vi "TC110.vi"(7 "Function":T3=enum."Read command", 8 "Error in":errorcluster, 10 "Settings in":T2) -> (0 "Error out":errorcluster, 1 "Status_string":string, 2 "Settings out":T2, 3 "output cluster":T1)   [LabVIEW 2018]
uses:
  clt/_ctl_PC_function_TC110.ctl
  clt/_ctl_PC_TurboSettings.ctl
  Public/Turbopumps/PV Operating adjustment - Cluster.ctl
  Pfeiffer Vacuum.lvlib
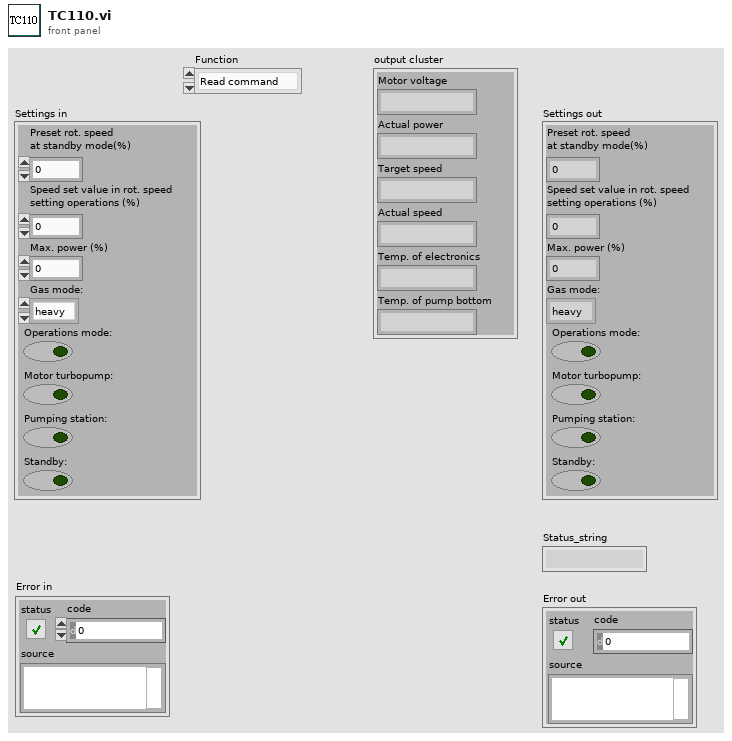
[diagram p1: front panel]
types:
  T1 = cluster{"Motor voltage":string, "Actual power":string, "Target speed":string, "Actual speed":string, "Temp. of electronics":string, "Temp. of pump bottom":string}
  T2 = typedef "_ctl_PC_TurboSettings.ctl" = cluster{"Preset rot. speed \nat standby mode(%)":dbl, "Speed set value in rot. speed \nsetting operations (%)":dbl, "Max. power (%)":dbl, "Gas mode: ":enum16{"heavy", "light", "helium"}, "Operations mode: ":bool, "Motor turbopump: ":bool, "Pumping station: ":bool, "Standby: ":bool}
  T3 = typedef "_ctl_PC_function_TC110.ctl" = enum16{"Initialisation", "Read status", "Write command", "Read command", "Close"}
  T4 = typedef "Pfeiffer Vacuum.lvlib/PV Operating adjustment - Cluster.ctl" = cluster{"Parameter":u16, "Parameter\nread only<->describe":bool, "off<->on":bool, "Rotation speed set value\nin rot. speed setting\noperations [%]":dbl, "Preset rotation Speed\nat Standby mode (%)":dbl, "maximum power\nsetpoint [%]":i32, "Gas mode":u16}
  T5 = enum16{"temperature inverter [°C] (324)", "temperature electronic [°C] (326)", "temperature pump bottom [°C] (330)", "temperature bearing [°C] (342)", "temperature motor [°C] (346)", "temperature rotor [°C] (384)"}
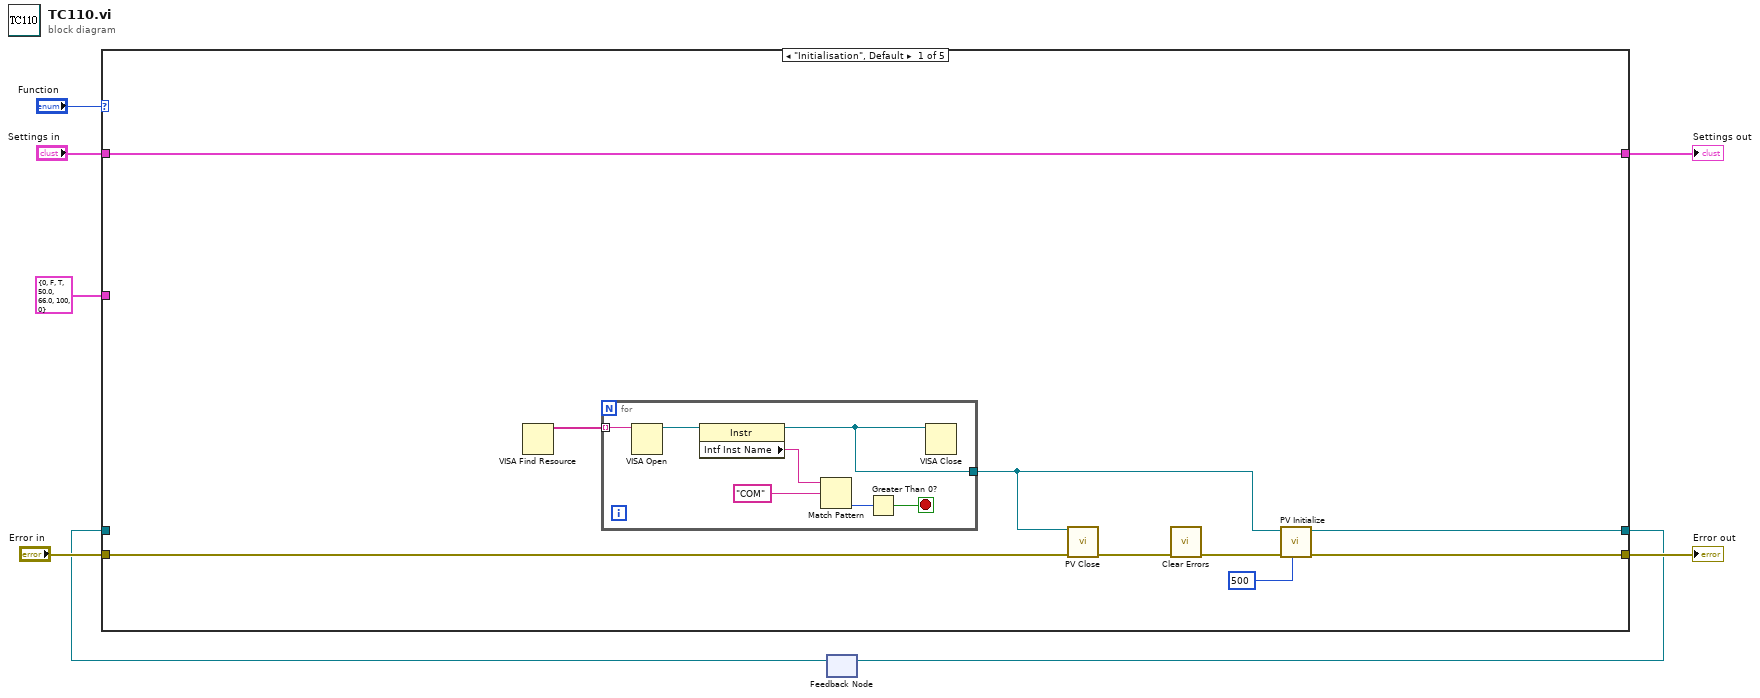
[diagram p0: block diagram]
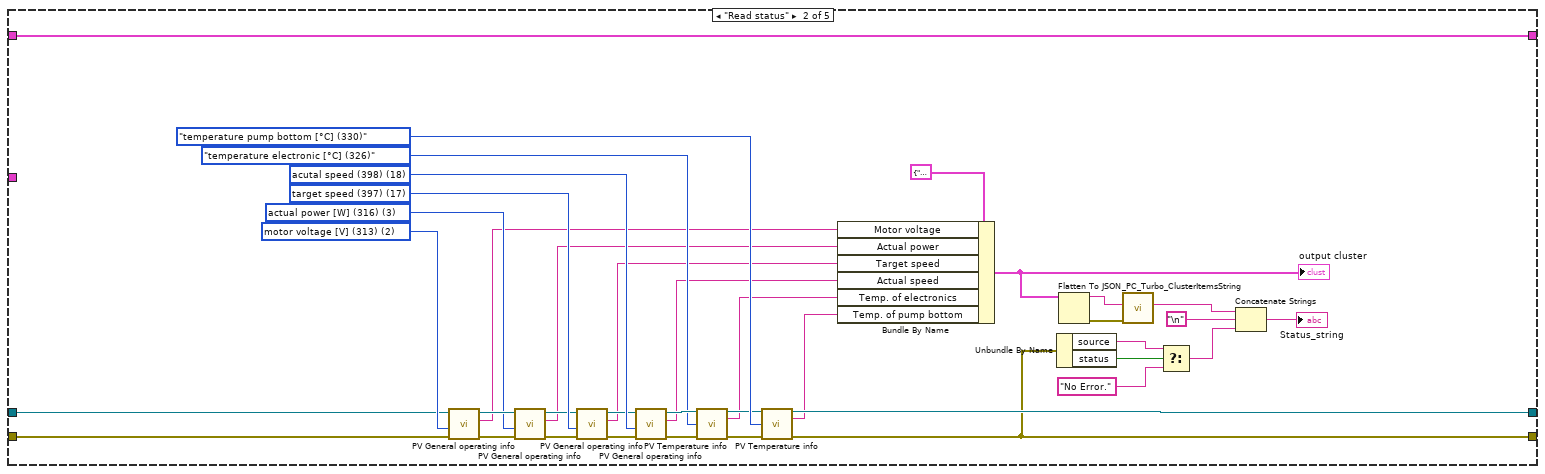
[diagram p2: hidden frame]
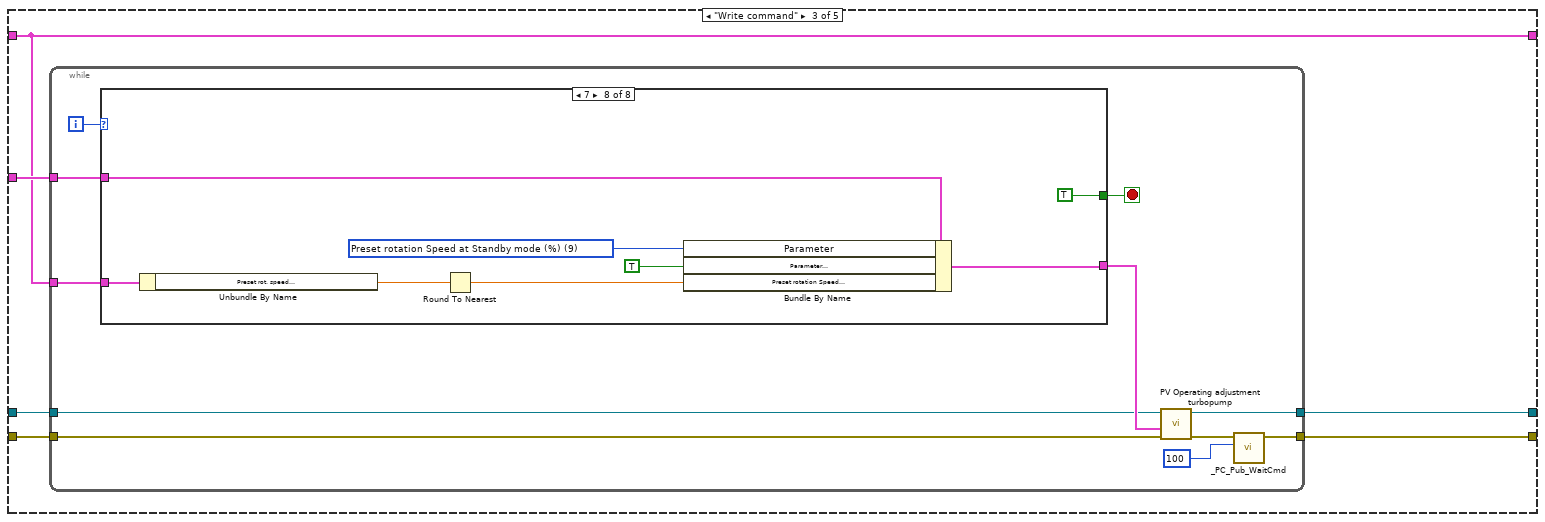
[diagram p3: hidden frame]
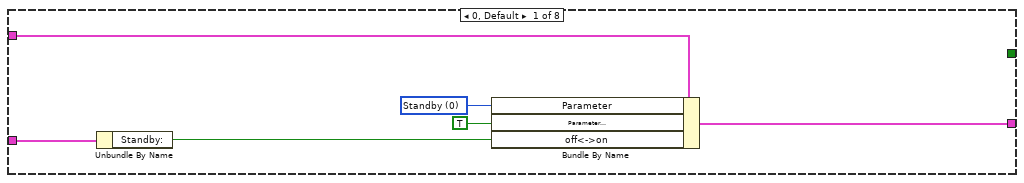
[diagram p4: hidden frame]
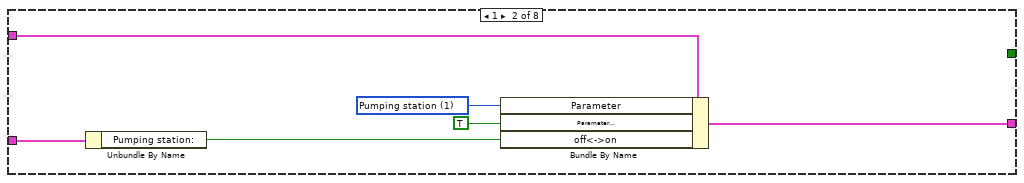
[diagram p5: hidden frame]
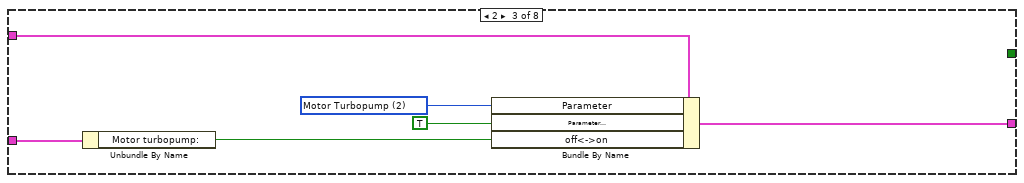
[diagram p6: hidden frame]
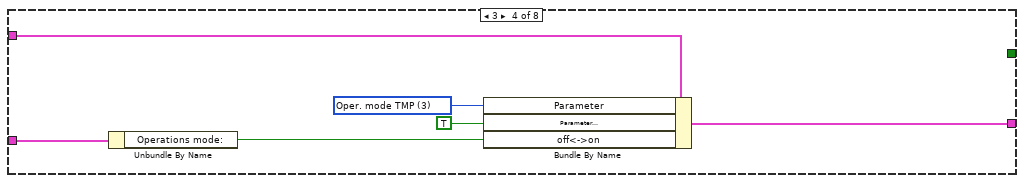
[diagram p7: hidden frame]
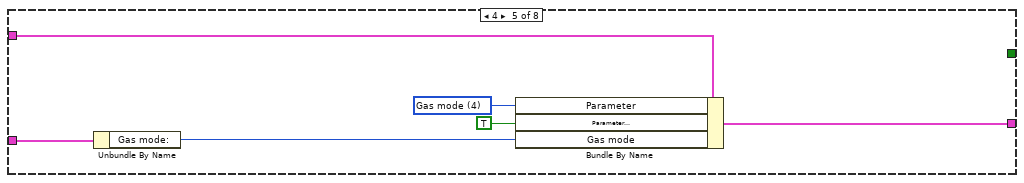
[diagram p8: hidden frame]
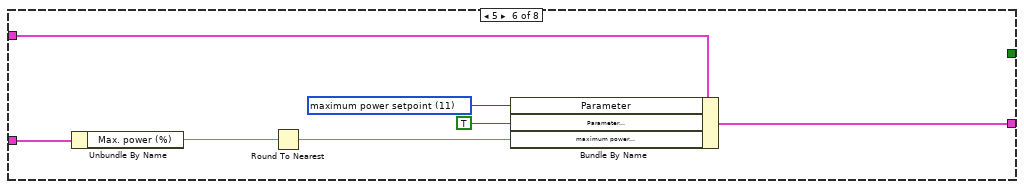
[diagram p9: hidden frame]
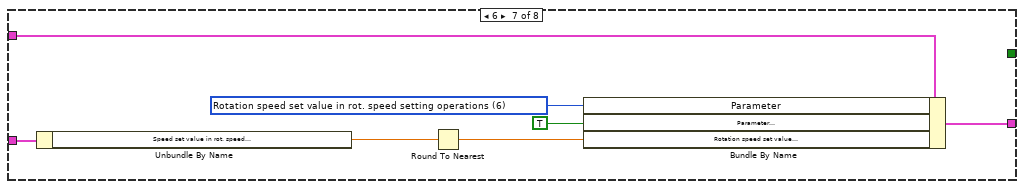
[diagram p10: hidden frame]
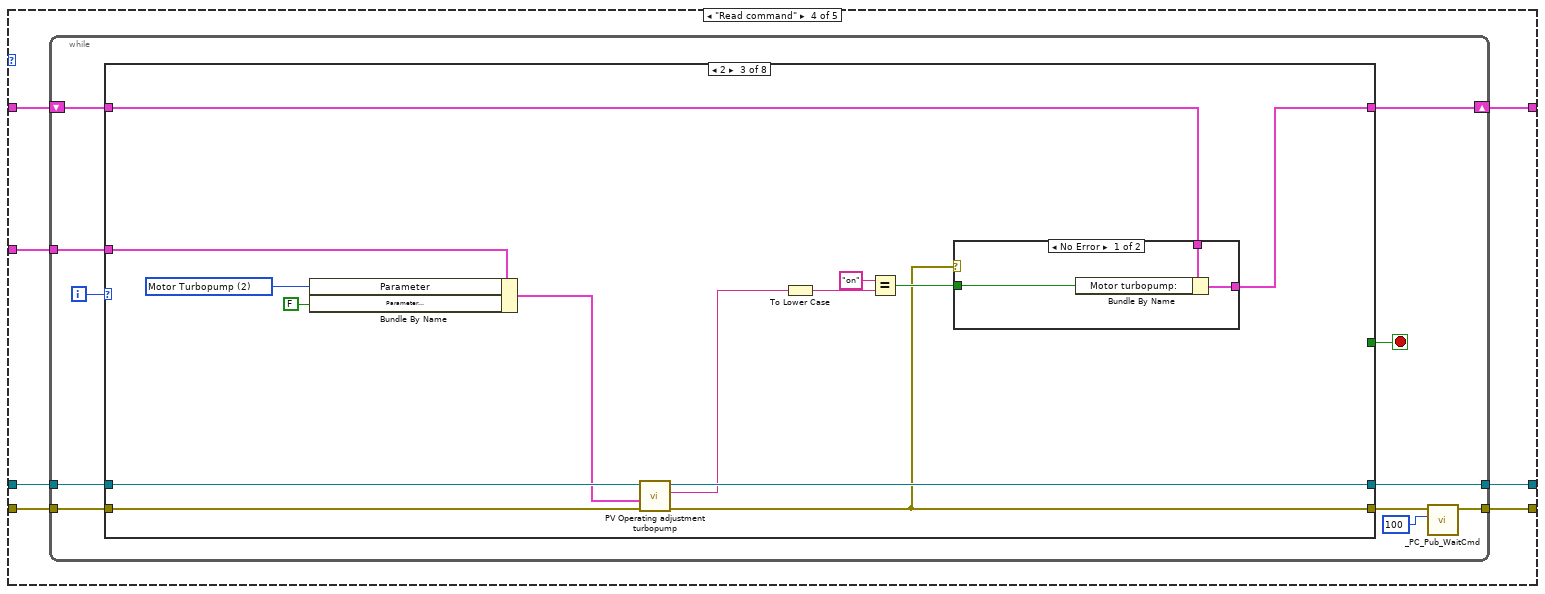
[diagram p11: hidden frame]
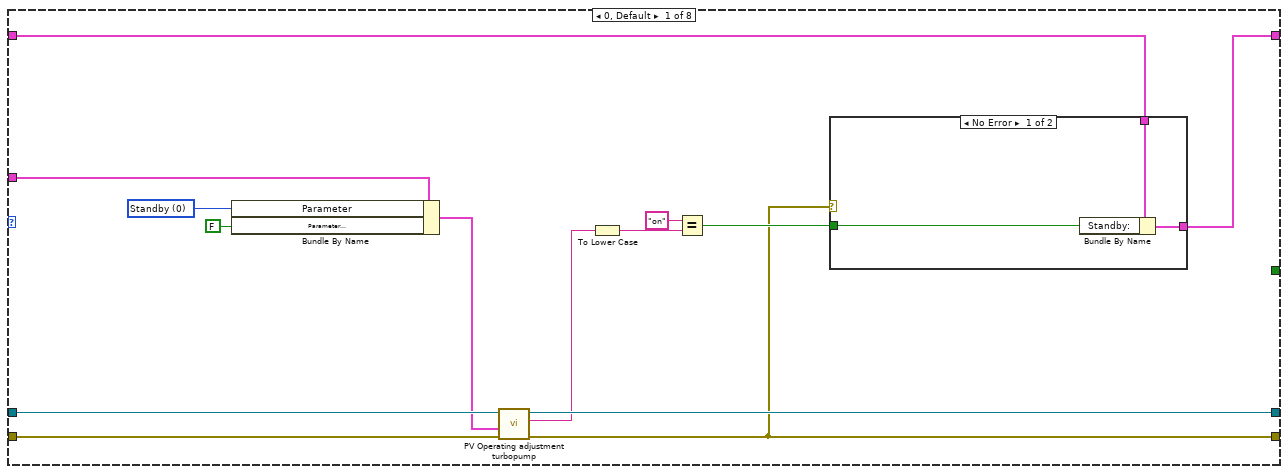
[diagram p12: hidden frame]
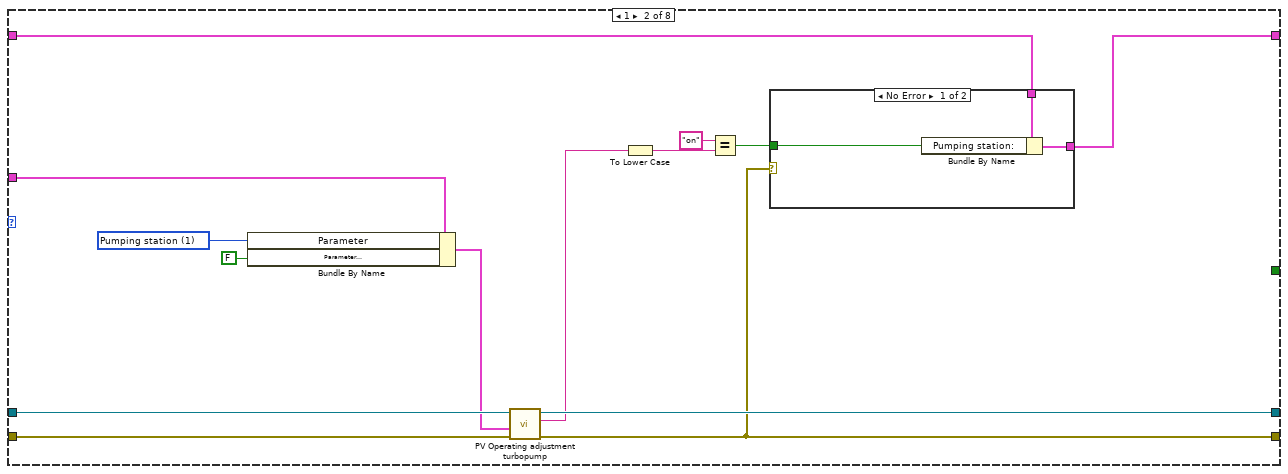
[diagram p14: hidden frame]
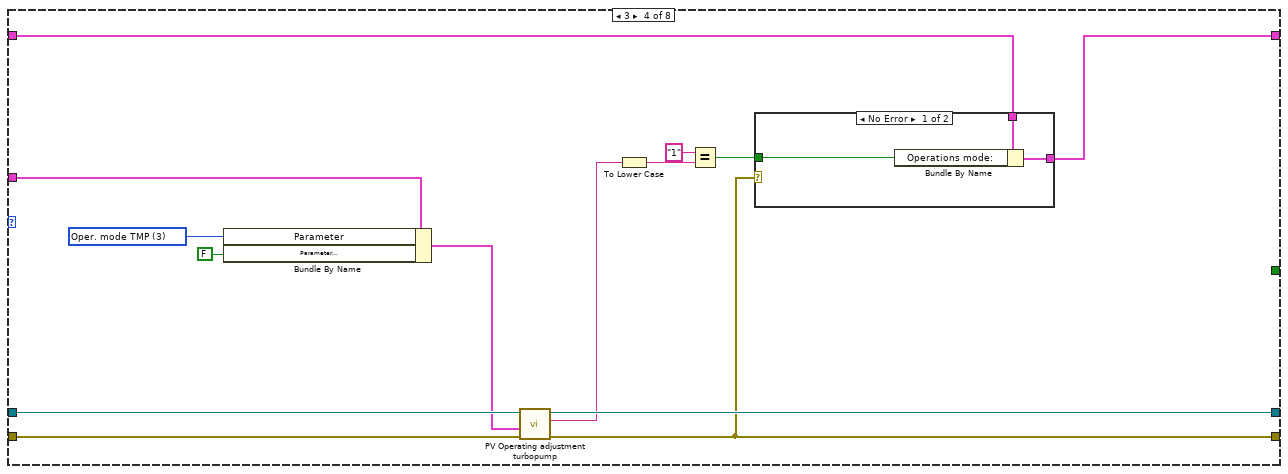
[diagram p17: hidden frame]
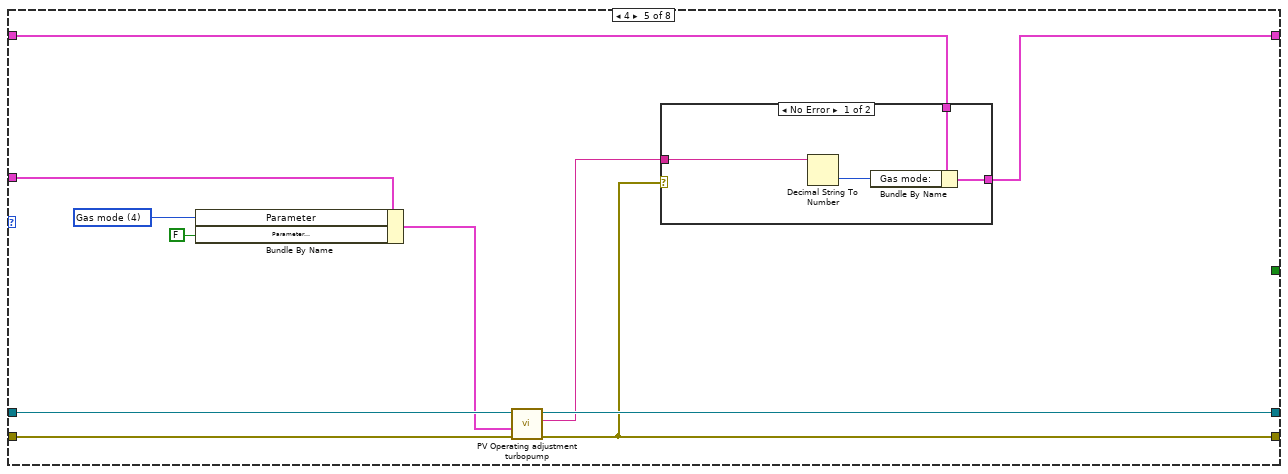
[diagram p19: hidden frame]
diagram:
  n1 = feedback #1() -> (w6:refnum<visa-resource-name>)  [unwired: 1 in]
  n2 = case shown="\"Initialisation\", Default" "Function" {
    tunnel: "Error in" -> [w13 w26 w66 w136 w291]
    tunnel: [w17 w42 w64 w133 _] -> w1
    tunnel: w6 -> [_ w27 w67 w137 w292]
    tunnel: [w16 w35 w65 w134 w290] -> w5
    tunnel: "Settings in" -> [w14 w25 w63 w135 w289]
    tunnel: T4 {"Parameter"=0, "Parameter\nread only<->describe"=FALSE, "off<->on"=TRUE, "Rotation speed set value\nin rot. speed setting\noperations [%]"=50.0, "Preset rotation Speed\nat Standby mode (%)"=66.0, "maximum power\nsetpoint [%]"=100, "Gas mode"=0} ("Operating adjustment - Cluster") -> [_ _ w68 w138 _]
    tunnel: [w14 w25 w63 w132 w289] -> w2
    frame "Initialisation", Default {
      n3 = VISA Find Resource() -> (3:w10:string[])  [unwired: 3 in, 2 out]
      n4 = for {
        tunnel: w10 -> [w24] mode=indexing
        tunnel: [w18] -> w9
        stop <- w20 stop-if-true
        n5 = VISA Open(VISA resource name=w24) -> (VISA resource name=w23:refnum<visa-resource-name>)  [unwired: 4 in, 1 out]
        n6 = property class="Instr"(reference=w23) -> (reference out=w18:refnum<visa-resource-name>, "Intf Inst Name"=w22:string)  [unwired: 1 in, 1 out]
        n7 = Match Pattern(string=w22, regular expression="COM") -> (offset past match=w19:i32)  [unwired: 1 in, 3 out]
        n8 = Greater Than 0?(x=w19) -> (x > 0?=w20:bool)
        n9 = VISA Close(VISA resource name=w18) -> ()  [unwired: 1 in, 1 out]
      }
      n10 = call "PV Close.vi"("VISA session"=w9, "error in (no error)"=w13) -> ("error out"=w12:errorcluster)  [unwired: 13 in]
      n11 = call <vilib>:"Clear Errors.vi"("error in (no error)"=w12) -> ("error out"=w11:errorcluster)  [unwired: 5 in, 1 out]
      n12 = call "PV Initialize.vi"("Timeout Value"=u32 500, "error in (no error)"=w11, "VISA session in"=w9) -> ("error out"=w16:errorcluster, "VISA session out"=w17:refnum<visa-resource-name>)  [unwired: 7 in]
    }
    frame "Read status" {
      w58 = u16 18 items=["nominal speed [Hz] (default) (315)", "intermediate circut current [A] (310)", "motor voltage [V] (313)", "actual power [W] (316)", "operating hours pump [h] (311)", "operating hours drive [h] (314)", "pump cycles (read only) (319)", "status oil sensor (read only) (301)", "speed switchpoint attained (read only) (302)", "overtemperature drive (read only) (304)", "overtemperature pump (read only) (305)", "target speed attained (read only) (306)", "pump accelerates (read only) (307) ", "controlled by remote (300)", "motor phase current [A] (317)", "acceleration / deceleration [rm/s] (336)", "hardware version controller (354)", "target speed (397)", "acutal speed (398)", "nominal speed (399)", "software version control unit (read only) (352)"] ("Parameter")
      w59 = u16 17 items=["nominal speed [Hz] (default) (315)", "intermediate circut current [A] (310)", "motor voltage [V] (313)", "actual power [W] (316)", "operating hours pump [h] (311)", "operating hours drive [h] (314)", "pump cycles (read only) (319)", "status oil sensor (read only) (301)", "speed switchpoint attained (read only) (302)", "overtemperature drive (read only) (304)", "overtemperature pump (read only) (305)", "target speed attained (read only) (306)", "pump accelerates (read only) (307) ", "controlled by remote (300)", "motor phase current [A] (317)", "acceleration / deceleration [rm/s] (336)", "hardware version controller (354)", "target speed (397)", "acutal speed (398)", "nominal speed (399)", "software version control unit (read only) (352)"] ("Parameter")
      w60 = u16 3 items=["nominal speed [Hz] (default) (315)", "intermediate circut current [A] (310)", "motor voltage [V] (313)", "actual power [W] (316)", "operating hours pump [h] (311)", "operating hours drive [h] (314)", "pump cycles (read only) (319)", "status oil sensor (read only) (301)", "speed switchpoint attained (read only) (302)", "overtemperature drive (read only) (304)", "overtemperature pump (read only) (305)", "target speed attained (read only) (306)", "pump accelerates (read only) (307) ", "controlled by remote (300)", "motor phase current [A] (317)", "acceleration / deceleration [rm/s] (336)", "hardware version controller (354)", "target speed (397)", "acutal speed (398)", "nominal speed (399)", "software version control unit (read only) (352)"] ("Parameter")
      w62 = u16 2 items=["nominal speed [Hz] (default) (315)", "intermediate circut current [A] (310)", "motor voltage [V] (313)", "actual power [W] (316)", "operating hours pump [h] (311)", "operating hours drive [h] (314)", "pump cycles (read only) (319)", "status oil sensor (read only) (301)", "speed switchpoint attained (read only) (302)", "overtemperature drive (read only) (304)", "overtemperature pump (read only) (305)", "target speed attained (read only) (306)", "pump accelerates (read only) (307) ", "controlled by remote (300)", "motor phase current [A] (317)", "acceleration / deceleration [rm/s] (336)", "hardware version controller (354)", "target speed (397)", "acutal speed (398)", "nominal speed (399)", "software version control unit (read only) (352)"] ("Parameter")
      n13 = call "PV General operating info.vi"("error in (no error)"=w26, "Parameter"=w62, "VISA session"=w27) -> ("error out"=w55:errorcluster, "response (data)"=w45:string, "dup VISA session"=w61:refnum<visa-resource-name>)  [unwired: 6 in]
      n14 = call "PV General operating info.vi"("error in (no error)"=w55, "Parameter"=w60, "VISA session"=w61) -> ("error out"=w54:errorcluster, "response (data)"=w39:string, "dup VISA session"=w57:refnum<visa-resource-name>)  [unwired: 6 in]
      n15 = call "PV General operating info.vi"("error in (no error)"=w54, "Parameter"=w59, "VISA session"=w57) -> ("error out"=w53:errorcluster, "response (data)"=w40:string, "dup VISA session"=w56:refnum<visa-resource-name>)  [unwired: 6 in]
      n16 = call "PV General operating info.vi"("error in (no error)"=w53, "Parameter"=w58, "VISA session"=w56) -> ("error out"=w49:errorcluster, "response (data)"=w44:string, "dup VISA session"=w52:refnum<visa-resource-name>)  [unwired: 6 in]
      n17 = call "PV Temperature info.vi"("VISA session"=w52, "Parameter"=T5."temperature electronic [°C] (326)", "error in (no error)"=w49) -> ("dup VISA session"=w48:refnum<visa-resource-name>, "response (data)"=w43:string, "error out"=w47:errorcluster)  [unwired: 10 in]
      n18 = call "PV Temperature info.vi"("VISA session"=w48, "Parameter"=T5."temperature pump bottom [°C] (330)", "error in (no error)"=w47) -> ("dup VISA session"=w42:refnum<visa-resource-name>, "response (data)"=w41:string, "error out"=w35:errorcluster)  [unwired: 10 in]
      n19 = Bundle By Name(cluster=T1 {"Motor voltage"="", "Actual power"="", "Target speed"="", "Actual speed"="", "Temp. of electronics"="", "Temp. of pump bottom"=""}, "Motor voltage"=w45, "Actual power"=w39, "Target speed"=w40, "Actual speed"=w44, "Temp. of electronics"=w43, "Temp. of pump bottom"=w41) -> (w38:T1)
      "output cluster" <- w38
      n20 = Unbundle By Name(w35) -> ("source"=w33:string, "status"=w34:bool)
      n21 = Flatten To JSON(anything=w38) -> (JSON string=w37:string, 11:w36:errorcluster)  [unwired: 2 in]
      n22 = call "_PC_Turbo_ClusterItemsString.vi"("error in (no error)"=w36, "JSON string"=w37) -> ("result string"=w31:string)  [unwired: 8 in, 1 out]
      n23 = Select(t=w33, s=w34, f="No Error.") -> (s? t:f=w29:string)
      n24 = Concatenate Strings(w31, "\n" ("string"), w29) -> (→"Status_string":string)
    }
    frame "Write command" {
      n25 = while {
        tunnel: w63 -> [w79]
        tunnel: w67 -> [w74]
        tunnel: w66 -> [w73]
        tunnel: [w70] -> w65
        tunnel: w68 -> [w78]
        tunnel: [w72] -> w64
        i -> [w77]
        stop <- w76 stop-if-true
        n26 = case shown="7" w77 {
          tunnel: w79 -> [w83 w89 w95 w101 w107 w114 w121 w129]
          tunnel: w78 -> [w85 w91 w97 w103 w109 w116 w123 w131]
          tunnel: [_ _ _ _ _ _ _ TRUE] -> w76
          tunnel: [w80 w86 w92 w98 w104 w110 w117 w124] -> w75
          frame 0, Default {
            w81 = u16 0 items=[" Standby", " Pumping station", " Motor Turbopump", " Oper. mode TMP", " Gas mode", " Operating mode drive unit", " Rotation speed set value in rot. speed setting operations", " Set rotation speed TMP [Hz] (read only)", " Actual rotation speed TMP [Hz] (read only)", " Preset rotation Speed at Standby mode (%)", " Max. rotations speed ", " maximum power setpoint"] ("Parameter")
            n27 = Unbundle By Name(w83) -> ("Standby:"=w82:bool)
            n28 = Bundle By Name(cluster=w85, "Parameter"=w81, "Parameter\nread only<->describe"=TRUE ("Parameter\nread only<->describe"), "off<->on"=w82) -> (w80:T4)
          }
          frame 1 {
            w87 = u16 1 items=[" Standby", " Pumping station", " Motor Turbopump", " Oper. mode TMP", " Gas mode", " Operating mode drive unit", " Rotation speed set value in rot. speed setting operations", " Set rotation speed TMP [Hz] (read only)", " Actual rotation speed TMP [Hz] (read only)", " Preset rotation Speed at Standby mode (%)", " Max. rotations speed ", " maximum power setpoint"] ("Parameter")
            n29 = Unbundle By Name(w89) -> ("Pumping station:"=w88:bool)
            n30 = Bundle By Name(cluster=w91, "Parameter"=w87, "Parameter\nread only<->describe"=TRUE ("Parameter\nread only<->describe"), "off<->on"=w88) -> (w86:T4)
          }
          frame 2 {
            w93 = u16 2 items=[" Standby", " Pumping station", " Motor Turbopump", " Oper. mode TMP", " Gas mode", " Operating mode drive unit", " Rotation speed set value in rot. speed setting operations", " Set rotation speed TMP [Hz] (read only)", " Actual rotation speed TMP [Hz] (read only)", " Preset rotation Speed at Standby mode (%)", " Max. rotations speed ", " maximum power setpoint"] ("Parameter")
            n31 = Unbundle By Name(w95) -> ("Motor turbopump:"=w94:bool)
            n32 = Bundle By Name(cluster=w97, "Parameter"=w93, "Parameter\nread only<->describe"=TRUE ("Parameter\nread only<->describe"), "off<->on"=w94) -> (w92:T4)
          }
          frame 3 {
            w99 = u16 3 items=[" Standby", " Pumping station", " Motor Turbopump", " Oper. mode TMP", " Gas mode", " Operating mode drive unit", " Rotation speed set value in rot. speed setting operations", " Set rotation speed TMP [Hz] (read only)", " Actual rotation speed TMP [Hz] (read only)", " Preset rotation Speed at Standby mode (%)", " Max. rotations speed ", " maximum power setpoint"] ("Parameter")
            n33 = Unbundle By Name(w101) -> ("Operations mode:"=w100:bool)
            n34 = Bundle By Name(cluster=w103, "Parameter"=w99, "Parameter\nread only<->describe"=TRUE ("Parameter\nread only<->describe"), "off<->on"=w100) -> (w98:T4)
          }
          frame 4 {
            w105 = u16 4 items=[" Standby", " Pumping station", " Motor Turbopump", " Oper. mode TMP", " Gas mode", " Operating mode drive unit", " Rotation speed set value in rot. speed setting operations", " Set rotation speed TMP [Hz] (read only)", " Actual rotation speed TMP [Hz] (read only)", " Preset rotation Speed at Standby mode (%)", " Max. rotations speed ", " maximum power setpoint"] ("Parameter")
            n35 = Unbundle By Name(w107) -> ("Gas mode:"=w106:enum16{"heavy", "light", "helium"})
            n36 = Bundle By Name(cluster=w109, "Parameter"=w105, "Parameter\nread only<->describe"=TRUE ("Parameter\nread only<->describe"), "Gas mode"=w106) -> (w104:T4)
          }
          frame 5 {
            w112 = u16 11 items=[" Standby", " Pumping station", " Motor Turbopump", " Oper. mode TMP", " Gas mode", " Operating mode drive unit", " Rotation speed set value in rot. speed setting operations", " Set rotation speed TMP [Hz] (read only)", " Actual rotation speed TMP [Hz] (read only)", " Preset rotation Speed at Standby mode (%)", " Max. rotations speed ", " maximum power setpoint"] ("Parameter")
            n37 = Unbundle By Name(w114) -> ("Max. power (%)"=w113:dbl)
            n38 = Round To Nearest(number=w113) -> (nearest integer value=w111:dbl)
            n39 = Bundle By Name(cluster=w116, "Parameter"=w112, "Parameter\nread only<->describe"=TRUE ("Parameter\nread only<->describe"), "maximum power\nsetpoint [%]"=w111) -> (w110:T4)
          }
          frame 6 {
            w119 = u16 6 items=[" Standby", " Pumping station", " Motor Turbopump", " Oper. mode TMP", " Gas mode", " Operating mode drive unit", " Rotation speed set value in rot. speed setting operations", " Set rotation speed TMP [Hz] (read only)", " Actual rotation speed TMP [Hz] (read only)", " Preset rotation Speed at Standby mode (%)", " Max. rotations speed ", " maximum power setpoint"] ("Parameter")
            n40 = Unbundle By Name(w121) -> ("Speed set value in rot. speed \nsetting operations (%)"=w120:dbl)
            n41 = Round To Nearest(number=w120) -> (nearest integer value=w118:dbl)
            n42 = Bundle By Name(cluster=w123, "Parameter"=w119, "Parameter\nread only<->describe"=TRUE ("Parameter\nread only<->describe"), "Rotation speed set value\nin rot. speed setting\noperations [%]"=w118) -> (w117:T4)
          }
          frame 7 {
            w127 = u16 9 items=[" Standby", " Pumping station", " Motor Turbopump", " Oper. mode TMP", " Gas mode", " Operating mode drive unit", " Rotation speed set value in rot. speed setting operations", " Set rotation speed TMP [Hz] (read only)", " Actual rotation speed TMP [Hz] (read only)", " Preset rotation Speed at Standby mode (%)", " Max. rotations speed ", " maximum power setpoint"] ("Parameter")
            n43 = Unbundle By Name(w129) -> ("Preset rot. speed \nat standby mode(%)"=w128:dbl)
            n44 = Round To Nearest(number=w128) -> (nearest integer value=w126:dbl)
            n45 = Bundle By Name(cluster=w131, "Parameter"=w127, "Parameter\nread only<->describe"=TRUE ("Parameter\nread only<->describe"), "Preset rotation Speed\nat Standby mode (%)"=w126) -> (w124:T4)
          }
        }
        n46 = call "PV Operating adjustment turbopump.vi"("error in (no error)"=w73, "Operating adjustment - Cluster"=w75, "VISA session"=w74) -> ("error out"=w71:errorcluster, "dup VISA session"=w72:refnum<visa-resource-name>)  [unwired: 6 in, 1 out]
        n47 = call "_PC_Pub_WaitCmd.vi"("milliseconds to wait"=u32 100, "error in (no error)"=w71) -> ("error out"=w70:errorcluster)  [unwired: 9 in]
      }
    }
    frame "Read command" {
      n48 = while {
        tunnel: w137 -> [w146]
        tunnel: w136 -> [w145]
        tunnel: [w147] -> w133
        tunnel: [w140] -> w134
        shift-right: [w143] -> w132
        shift-left: w135 -> [w142]
        tunnel: w138 -> [w149]
        i -> [w148]
        stop <- w144 stop-if-true
        n49 = case shown="2" w148 {
          tunnel: w149 -> [w154 w181 w199 w217 w232 w248 w264 w281]
          tunnel: [w162 w179 w197 w215 w230 w246 w262 w279] -> w147
          tunnel: w146 -> [w161 w178 w196 w214 w229 w245 w261 w278]
          tunnel: [w151 w168 w188 w207 w224 w240 w257 w273] -> w141
          tunnel: w145 -> [w159 w176 w194 w212 w227 w244 w259 w277]
          tunnel: [_ _ _ _ _ _ _ TRUE] -> w144
          tunnel: [w152 w171 w186 w204 w222 w238 w254 w270] -> w143
          tunnel: w142 -> [w150 w169 w187 w205 w223 w239 w255 w271]
          frame 0, Default {
            w158 = u16 0 items=[" Standby", " Pumping station", " Motor Turbopump", " Oper. mode TMP", " Gas mode", " Operating mode drive unit", " Rotation speed set value in rot. speed setting operations", " Set rotation speed TMP [Hz] (read only)", " Actual rotation speed TMP [Hz] (read only)", " Preset rotation Speed at Standby mode (%)", " Max. rotations speed ", " maximum power setpoint"] ("Parameter")
            n50 = Bundle By Name(cluster=w154, "Parameter"=w158, "Parameter\nread only<->describe"=FALSE ("Parameter\nread only<->describe")) -> (w160:T4)
            n51 = call "PV Operating adjustment turbopump.vi"("error in (no error)"=w159, "Operating adjustment - Cluster"=w160, "VISA session"=w161) -> ("error out"=w151:errorcluster, "response (data)"=w155:string, "dup VISA session"=w162:refnum<visa-resource-name>)  [unwired: 6 in]
            n52 = To Lower Case(string=w155) -> (all lower case string=w156:string)
            n53 = Equal?(x="on", y=w156) -> (x = y?=w153:bool)
            n54 = case shown="No Error" w151 {
              tunnel: w153 -> [w166 _]
              tunnel: [w165 w167] -> w152
              tunnel: w150 -> [w164 w167]
              frame No Error {
                n55 = Bundle By Name(cluster=w164, "Standby:"=w166) -> (w165:T2)
              }
              frame Error {
              }
            }
          }
          frame 1 {
            w175 = u16 1 items=[" Standby", " Pumping station", " Motor Turbopump", " Oper. mode TMP", " Gas mode", " Operating mode drive unit", " Rotation speed set value in rot. speed setting operations", " Set rotation speed TMP [Hz] (read only)", " Actual rotation speed TMP [Hz] (read only)", " Preset rotation Speed at Standby mode (%)", " Max. rotations speed ", " maximum power setpoint"] ("Parameter")
            n56 = Bundle By Name(cluster=w181, "Parameter"=w175, "Parameter\nread only<->describe"=FALSE ("Parameter\nread only<->describe")) -> (w177:T4)
            n57 = call "PV Operating adjustment turbopump.vi"("error in (no error)"=w176, "Operating adjustment - Cluster"=w177, "VISA session"=w178) -> ("error out"=w168:errorcluster, "response (data)"=w170:string, "dup VISA session"=w179:refnum<visa-resource-name>)  [unwired: 6 in]
            n58 = To Lower Case(string=w170) -> (all lower case string=w173:string)
            n59 = Equal?(x="on", y=w173) -> (x = y?=w172:bool)
            n60 = case shown="No Error" w168 {
              tunnel: w172 -> [w184 _]
              tunnel: [w183 w185] -> w171
              tunnel: w169 -> [w182 w185]
              frame No Error {
                n61 = Bundle By Name(cluster=w182, "Pumping station:"=w184) -> (w183:T2)
              }
              frame Error {
              }
            }
          }
          frame 2 {
            w193 = u16 2 items=[" Standby", " Pumping station", " Motor Turbopump", " Oper. mode TMP", " Gas mode", " Operating mode drive unit", " Rotation speed set value in rot. speed setting operations", " Set rotation speed TMP [Hz] (read only)", " Actual rotation speed TMP [Hz] (read only)", " Preset rotation Speed at Standby mode (%)", " Max. rotations speed ", " maximum power setpoint"] ("Parameter")
            n62 = Bundle By Name(cluster=w199, "Parameter"=w193, "Parameter\nread only<->describe"=FALSE ("Parameter\nread only<->describe")) -> (w195:T4)
            n63 = call "PV Operating adjustment turbopump.vi"("error in (no error)"=w194, "Operating adjustment - Cluster"=w195, "VISA session"=w196) -> ("error out"=w188:errorcluster, "response (data)"=w189:string, "dup VISA session"=w197:refnum<visa-resource-name>)  [unwired: 6 in]
            n64 = To Lower Case(string=w189) -> (all lower case string=w191:string)
            n65 = Equal?(x="on", y=w191) -> (x = y?=w190:bool)
            n66 = case shown="No Error" w188 {
              tunnel: w190 -> [w202 _]
              tunnel: [w201 w203] -> w186
              tunnel: w187 -> [w200 w203]
              frame No Error {
                n67 = Bundle By Name(cluster=w200, "Motor turbopump:"=w202) -> (w201:T2)
              }
              frame Error {
              }
            }
          }
          frame 3 {
            w211 = u16 3 items=[" Standby", " Pumping station", " Motor Turbopump", " Oper. mode TMP", " Gas mode", " Operating mode drive unit", " Rotation speed set value in rot. speed setting operations", " Set rotation speed TMP [Hz] (read only)", " Actual rotation speed TMP [Hz] (read only)", " Preset rotation Speed at Standby mode (%)", " Max. rotations speed ", " maximum power setpoint"] ("Parameter")
            n68 = Bundle By Name(cluster=w217, "Parameter"=w211, "Parameter\nread only<->describe"=FALSE ("Parameter\nread only<->describe")) -> (w213:T4)
            n69 = call "PV Operating adjustment turbopump.vi"("error in (no error)"=w212, "Operating adjustment - Cluster"=w213, "VISA session"=w214) -> ("error out"=w207:errorcluster, "response (data)"=w208:string, "dup VISA session"=w215:refnum<visa-resource-name>)  [unwired: 6 in]
            n70 = To Lower Case(string=w208) -> (all lower case string=w210:string)
            n71 = Equal?(x="1", y=w210) -> (x = y?=w209:bool)
            n72 = case shown="No Error" w207 {
              tunnel: w209 -> [w220 _]
              tunnel: [w219 w221] -> w204
              tunnel: w205 -> [w218 w221]
              frame No Error {
                n73 = Bundle By Name(cluster=w218, "Operations mode:"=w220) -> (w219:T2)
              }
              frame Error {
              }
            }
          }
          frame 4 {
            w226 = u16 4 items=[" Standby", " Pumping station", " Motor Turbopump", " Oper. mode TMP", " Gas mode", " Operating mode drive unit", " Rotation speed set value in rot. speed setting operations", " Set rotation speed TMP [Hz] (read only)", " Actual rotation speed TMP [Hz] (read only)", " Preset rotation Speed at Standby mode (%)", " Max. rotations speed ", " maximum power setpoint"] ("Parameter")
            n74 = Bundle By Name(cluster=w232, "Parameter"=w226, "Parameter\nread only<->describe"=FALSE ("Parameter\nread only<->describe")) -> (w228:T4)
            n75 = call "PV Operating adjustment turbopump.vi"("error in (no error)"=w227, "Operating adjustment - Cluster"=w228, "VISA session"=w229) -> ("error out"=w224:errorcluster, "response (data)"=w225:string, "dup VISA session"=w230:refnum<visa-resource-name>)  [unwired: 6 in]
            n76 = case shown="No Error" w224 {
              tunnel: w225 -> [w236 _]
              tunnel: w223 -> [w234 w237]
              tunnel: [w233 w237] -> w222
              frame No Error {
                n77 = Decimal String To Number(string=w236) -> (number=w235:i32)  [unwired: 2 in, 1 out]
                n78 = Bundle By Name(cluster=w234, "Gas mode:"=w235) -> (w233:T2)
              }
              frame Error {
              }
            }
          }
          frame 5 {
            w243 = u16 11 items=[" Standby", " Pumping station", " Motor Turbopump", " Oper. mode TMP", " Gas mode", " Operating mode drive unit", " Rotation speed set value in rot. speed setting operations", " Set rotation speed TMP [Hz] (read only)", " Actual rotation speed TMP [Hz] (read only)", " Preset rotation Speed at Standby mode (%)", " Max. rotations speed ", " maximum power setpoint"] ("Parameter")
            n79 = Bundle By Name(cluster=w248, "Parameter"=w243, "Parameter\nread only<->describe"=FALSE ("Parameter\nread only<->describe")) -> (w242:T4)
            n80 = call "PV Operating adjustment turbopump.vi"("error in (no error)"=w244, "Operating adjustment - Cluster"=w242, "VISA session"=w245) -> ("error out"=w240:errorcluster, "response (data)"=w241:string, "dup VISA session"=w246:refnum<visa-resource-name>)  [unwired: 6 in]
            n81 = case shown="No Error" w240 {
              tunnel: w241 -> [w251 _]
              tunnel: w239 -> [w250 w253]
              tunnel: [w249 w253] -> w238
              frame No Error {
                n82 = Fract/Exp String To Number(string=w251) -> (number=w252:dbl)  [unwired: 3 in, 1 out]
                n83 = Bundle By Name(cluster=w250, "Max. power (%)"=w252) -> (w249:T2)
              }
              frame Error {
              }
            }
          }
          frame 6 {
            w258 = u16 6 items=[" Standby", " Pumping station", " Motor Turbopump", " Oper. mode TMP", " Gas mode", " Operating mode drive unit", " Rotation speed set value in rot. speed setting operations", " Set rotation speed TMP [Hz] (read only)", " Actual rotation speed TMP [Hz] (read only)", " Preset rotation Speed at Standby mode (%)", " Max. rotations speed ", " maximum power setpoint"] ("Parameter")
            n84 = Bundle By Name(cluster=w264, "Parameter"=w258, "Parameter\nread only<->describe"=FALSE ("Parameter\nread only<->describe")) -> (w260:T4)
            n85 = call "PV Operating adjustment turbopump.vi"("error in (no error)"=w259, "Operating adjustment - Cluster"=w260, "VISA session"=w261) -> ("error out"=w257:errorcluster, "response (data)"=w256:string, "dup VISA session"=w262:refnum<visa-resource-name>)  [unwired: 6 in]
            n86 = case shown="No Error" w257 {
              tunnel: w256 -> [w267 _]
              tunnel: [w266 w269] -> w254
              tunnel: w255 -> [w265 w269]
              frame No Error {
                n87 = Fract/Exp String To Number(string=w267) -> (number=w268:dbl)  [unwired: 3 in, 1 out]
                n88 = Bundle By Name(cluster=w265, "Speed set value in rot. speed \nsetting operations (%)"=w268) -> (w266:T2)
              }
              frame Error {
              }
            }
          }
          frame 7 {
            w276 = u16 9 items=[" Standby", " Pumping station", " Motor Turbopump", " Oper. mode TMP", " Gas mode", " Operating mode drive unit", " Rotation speed set value in rot. speed setting operations", " Set rotation speed TMP [Hz] (read only)", " Actual rotation speed TMP [Hz] (read only)", " Preset rotation Speed at Standby mode (%)", " Max. rotations speed ", " maximum power setpoint"] ("Parameter")
            n89 = Bundle By Name(cluster=w281, "Parameter"=w276, "Parameter\nread only<->describe"=FALSE ("Parameter\nread only<->describe")) -> (w275:T4)
            n90 = call "PV Operating adjustment turbopump.vi"("error in (no error)"=w277, "Operating adjustment - Cluster"=w275, "VISA session"=w278) -> ("error out"=w273:errorcluster, "response (data)"=w272:string, "dup VISA session"=w279:refnum<visa-resource-name>)  [unwired: 6 in]
            n91 = case shown="No Error" w273 {
              tunnel: [w284 w288] -> w270
              tunnel: w272 -> [w283 _]
              tunnel: w271 -> [w282 w288]
              frame No Error {
                n92 = Fract/Exp String To Number(string=w283) -> (number=w287:dbl)  [unwired: 3 in, 1 out]
                n93 = Divide(x=w287, y=100.0) -> (x/y=w286:dbl)
                n94 = Bundle By Name(cluster=w282, "Preset rot. speed \nat standby mode(%)"=w286) -> (w284:T2)
              }
              frame Error {
              }
            }
          }
        }
        n95 = call "_PC_Pub_WaitCmd.vi"("milliseconds to wait"=u32 100, "error in (no error)"=w141) -> ("error out"=w140:errorcluster)  [unwired: 9 in]
      }
    }
    frame "Close" {
      n96 = call "PV Close.vi"("VISA session"=w292, "error in (no error)"=w291) -> ("error out"=w290:errorcluster)  [unwired: 13 in]
    }
  }
  "Error out" <- w5
  "Settings out" <- w2
  n97 = feedback-in #1(w1) -> ()
